vi "Event Handler.vi"(0 "uService Template in":refnum<class "Detector Manager.lvclass">, 5 "Event type":T1=enum."Message", 7 "Item Name":string, 9 "Data":variant, 11 "error in (no error)":errorcluster) -> (4 "uService Template out":refnum<class "Detector Manager.lvclass">, 15 "error out":errorcluster)   [LabVIEW 2026, in "TALOS.lvlib" / "Detector Manager.lvlib" / "Detector Manager.lvclass"]
uses:
  Detector Manager.lvclass
  C:/LabVIEW Code/TALOS/talos/Father of all uServices/Father of all uServices/Father of all uServices.lvclass
  Father of all uServices/Father of all uServices/Event Handler Items.ctl
  Ancestor/Ancestor/Ancestor.lvclass/Ancestor.ctl
  Detector Manager Consumer Case Selector.ctl
  Detector Manager.lvclass/Detector Manager.ctl
  Father of all uServices/Father of all uServices Messages/Consumer Msg/Consumer Msg.lvclass/Consumer Msg.ctl
  FGV/Error Memory/Get Error Description.vi
  Support VIs/Get PC name.vi
  Ancestor/Ancestor/Read ID.vi
  Support VIs/Get Class Name.vi
  <vilib>/Utility/error.llb/Clear Errors.vi
  Father of all uServices/Father of all uServices Messages/Consumer Msg/Send Consumer.vi
  FGV/Error Memory/Error Memory Core.vi
  <vilib>/AdvancedString/Delimited String to 1D String Array.vi
  <vilib>/AdvancedString/Delimited String to 1D String Array (string).vi
  Support VIs/Circus Root Path.vi
  FGV/Error Memory/Error Crt Lvl checker.vi
  FGV/Error Memory/Error Memory Core.vi/40c8088d-b597-4017-91af-faa98e00292e.vi
  FGV/Error Memory/Error Memory Core.vi/d4a3ab98-063c-4e44-b43d-fbdcfe6c2be2.vi
  Father of all uServices/Father of all uServices/Father of all uServices.lvclass
  C:/LabVIEW Code/TALOS/builds/Actor Framework PPL/Actor Framework.lvlibp/1abvi3w/vi.lib/ActorFramework/Actor/Actor.lvclass
  Support VIs/Global Memory.vi
  <vilib>/Utility/LVClass/Get LV Class Name.vi
  Support VIs/Is in Packed Library.vi
  Support VIs/TALOS Root path.vi
  Support VIs/Read CSV worksheet.vi
  Support VIs/Global Constants.vi
  <vilib>/Utility/error.llb/General Error Handler.vi
  builds/Actor Framework PPL/Actor Framework.lvlibp/1abvi3w/vi.lib/ActorFramework/Actor/Read Self Enqueuer.vi
  <userlib>/_OpenG.lib/lvdata/lvdata.llb/Get Strings from Enum__ogtk.vi
  builds/Actor Framework PPL/Actor Framework.lvlibp/1abvi3w/vi.lib/ActorFramework/Message Enqueuer/Enqueue.vi
  Support VIs/Error Log.vi
  Ancestor/Ancestor/Ancestor.lvclass
  <vilib>/Comparison/Equal/Equal Functor/Equal Functor.lvclass
  Father of all uServices/Father of all uServices Messages/Consumer Msg/Consumer Msg.lvclass
  Classes/Father of all Detectors/Father Of All Detectors.lvclass
  TALOS.lvlib
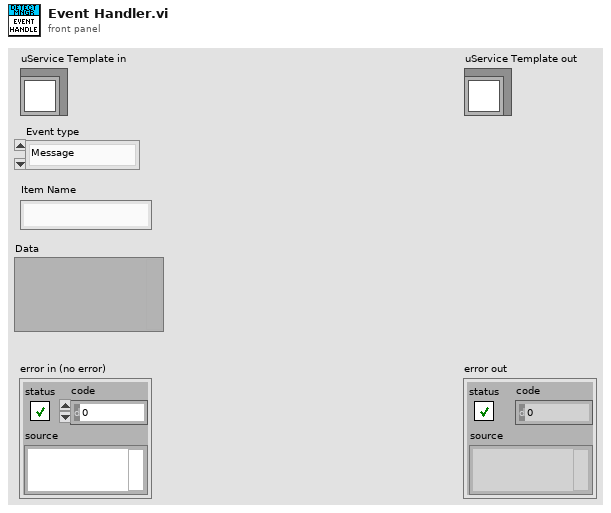
[diagram p1: front panel]
types:
  T1 = typedef "TALOS.lvlib/Father of all uServices.lvlib/Father of all uServices.lvclass/Event Handler Items.ctl" = enum16{"Button Pressed", "Message", "Ready to launch?", "Safe Mode", "Start RUN", "Stop RUN"}
  T2 = typedef "TALOS.lvlib/Detector Manager.lvlib/Detector Manager.lvclass/Detector Manager Consumer Case Selector.ctl" = enum16{"Set Configuration", "Arm", "Acquiring", "Save Data", "Self Check", "Safe Mode", "Init", "Close", "Stop"}
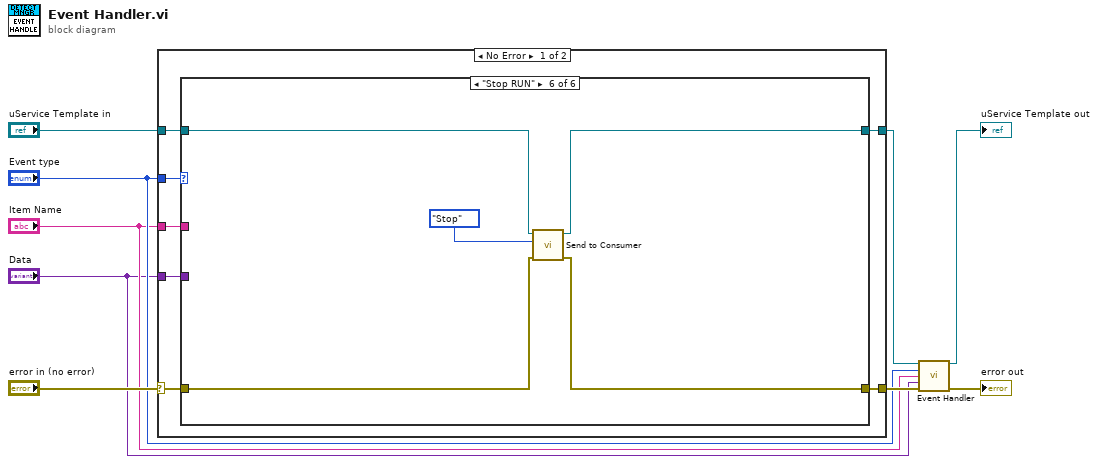
[diagram p0: block diagram]
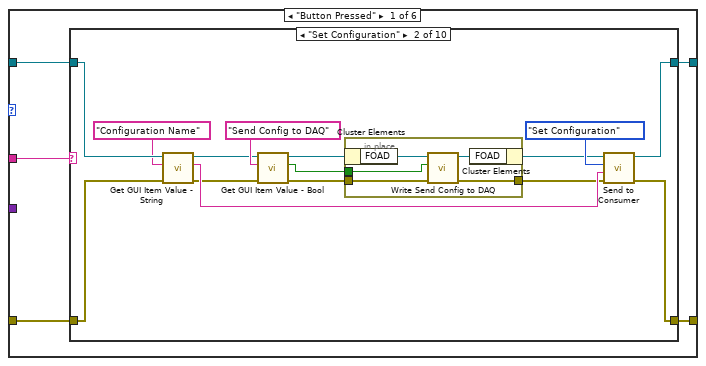
[diagram p2: hidden frame]
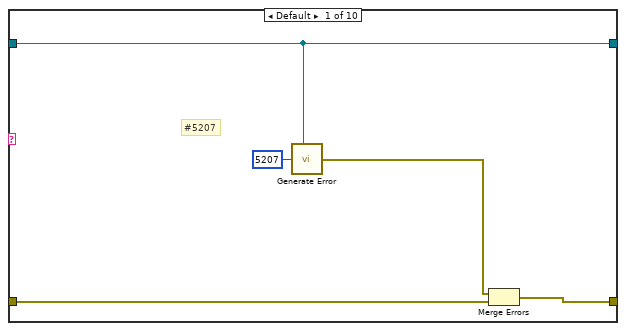
[diagram p3: hidden frame]
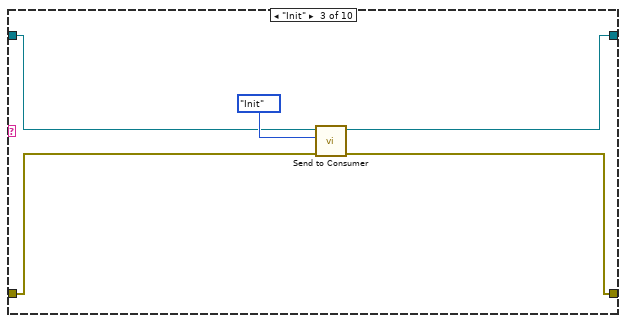
[diagram p4: hidden frame]
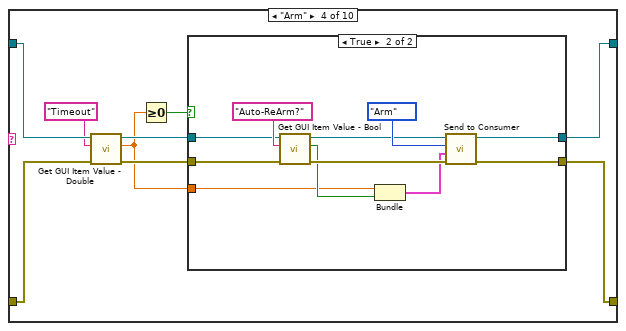
[diagram p5: hidden frame]
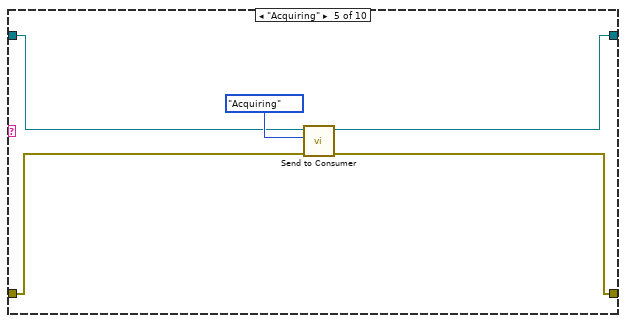
[diagram p7: hidden frame]
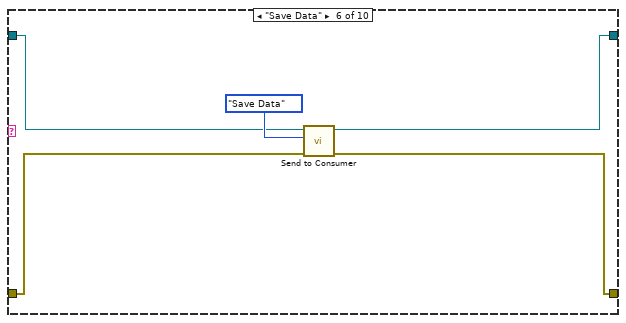
[diagram p8: hidden frame]
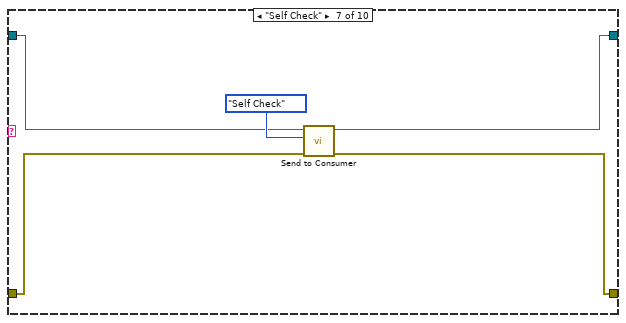
[diagram p9: hidden frame]
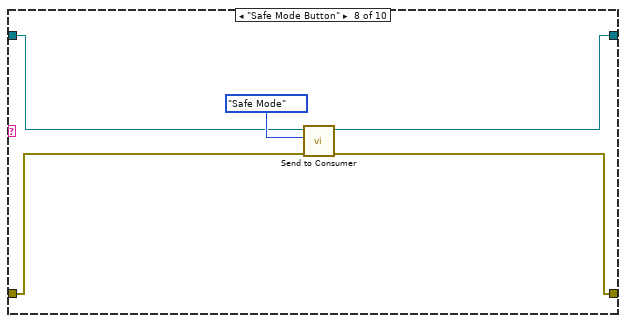
[diagram p10: hidden frame]
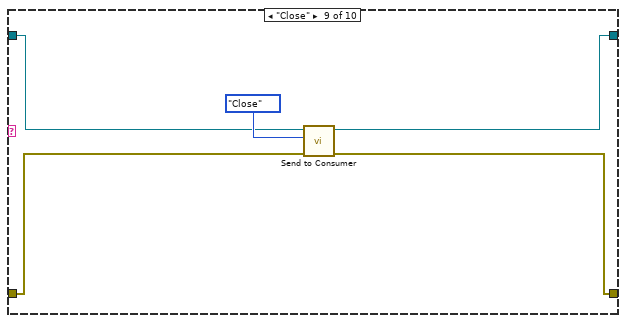
[diagram p11: hidden frame]
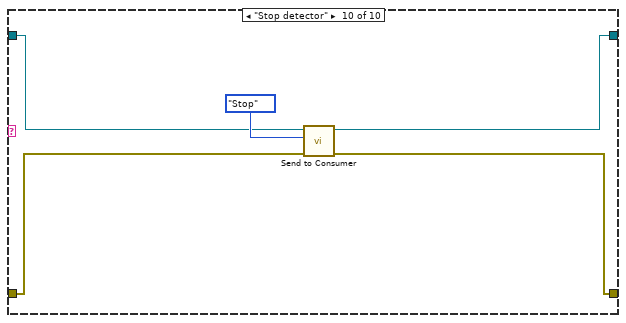
[diagram p12: hidden frame]
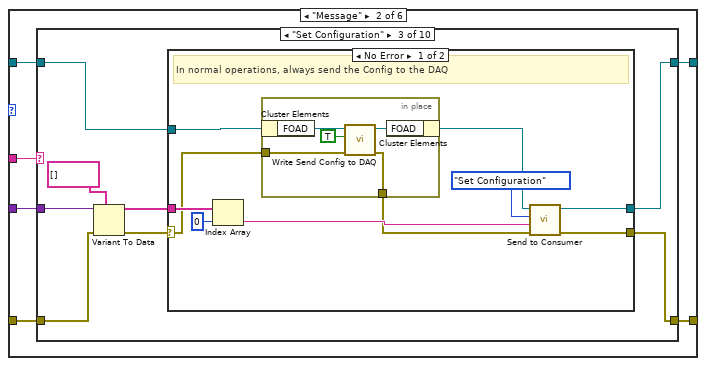
[diagram p13: hidden frame]
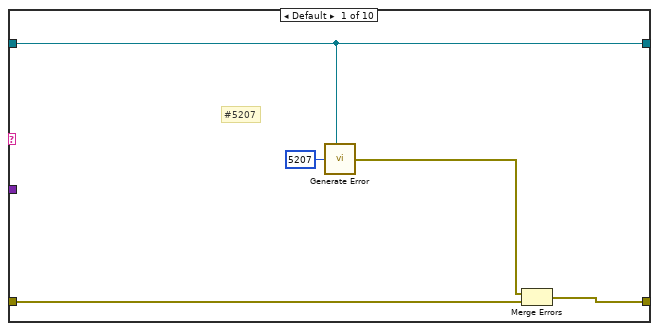
[diagram p14: hidden frame]
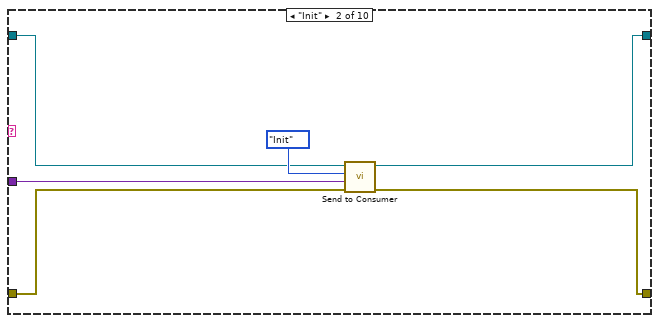
[diagram p15: hidden frame]
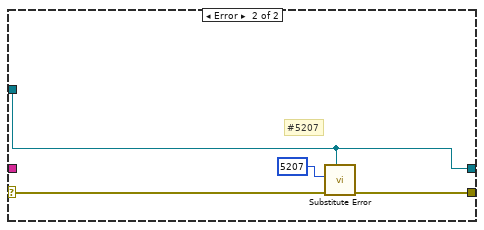
[diagram p16: hidden frame]
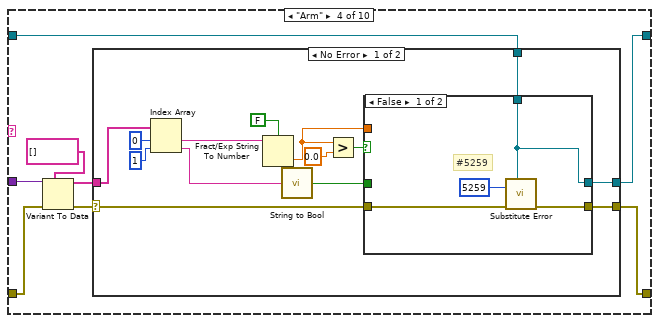
[diagram p17: hidden frame]
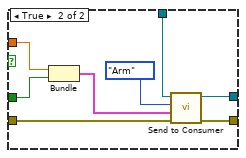
[diagram p18: hidden frame]
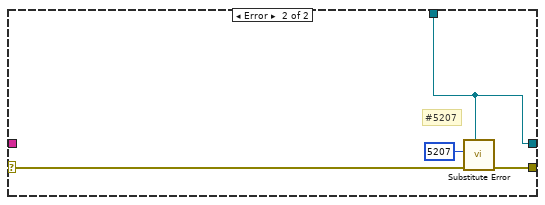
[diagram p19: hidden frame]
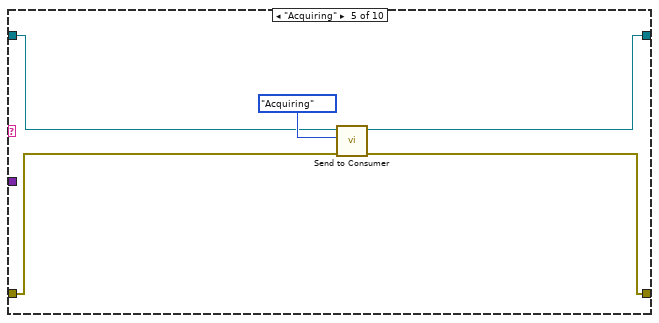
[diagram p20: hidden frame]
diagram:
  n1 = case shown="No Error" "error in (no error)" {
    selector: "error in (no error)" -> [w13 w235]
    tunnel: [w12 w235] -> w7
    tunnel: "uService Template in" -> [w15 w234]
    tunnel: [w14 w234] -> w4
    tunnel: "Event type" -> [w16 _]
    tunnel: "Item Name" -> [w11 _]
    tunnel: "Data" -> [w10 _]
    frame No Error {
      n2 = case shown="\"Stop RUN\"" w16 {
        tunnel: w15 -> [w21 w109 w220 w224 w228 w232]
        tunnel: [w20 w108 w219 w225 w228 w229] -> w14
        tunnel: w13 -> [w17 w105 w218 w222 w227 w231]
        tunnel: [w18 w106 w217 w223 w227 w230] -> w12
        tunnel: w11 -> [w19 w107 _ _ _ _]
        tunnel: w10 -> [_ w104 w216 _ _ _]
        frame "Button Pressed" {
          n3 = case shown="\"Set Configuration\"" w19 {
            tunnel: w21 -> [w22 w40 w50 w60 w77 w82 w87 w92 w97 w102]
            tunnel: [w22 w39 w49 w59 w76 w81 w86 w91 w96 w101] -> w20
            tunnel: [w25 w38 w48 w58 w75 w80 w85 w90 w95 w100] -> w18
            tunnel: w17 -> [w26 w37 w47 w57 w74 w79 w84 w89 w94 w99]
            frame Default {
              # "#5207"
              n4 = call "Generate Error.vi"("Class"=w22, "Error Code"=5207) -> ("error out"=w24:errorcluster)  [unwired: 5 in]
              n5 = Merge Errors(w24, w26) -> (w25:errorcluster)
            }
            frame "Set Configuration" {
              n6 = call "Get GUI Item Value - String.vi"("error in (no error)"=w37, "FP Item Name"="Configuration Name", "uService Template in"=w40) -> ("error out"=w33:errorcluster, "Value"=w35:string, "uService Template out"=w32:refnum<class "Detector Manager.lvclass">)  [unwired: 6 in]
              n7 = call "Get GUI Item Value - Bool.vi"("error in (no error)"=w33, "FP Item Name"="Send Config to DAQ", "uService Template in"=w32) -> ("error out"=w31:errorcluster, "Value"=w29:bool, "uService Template out"=w28:refnum<class "Detector Manager.lvclass">)  [unwired: 6 in]
              n8 = in-place {
                in-place-border: w31 -> [w44]
                in-place-border: [w43] -> w30
                in-place-border: w29 -> [w42]
                n9 = in-place-cluster #1(w28) -> ("FOAD"=w46:refnum<class "Father Of All Detectors.lvclass">)
                n10 = call-dynamic "Write Send Config to DAQ.vi"("error in (no error)"=w44, "Send Config to DAQ"=w42, "Father Of All Detectors in"=w46) -> ("error out"=w43:errorcluster, "Father Of All Detectors out"=w45:refnum<class "Father Of All Detectors.lvclass">)  [unwired: 7 in]
                n11 = in-place-cluster #1("FOAD"=w45) -> (w27:refnum<class "Detector Manager.lvclass">)
              }
              n12 = call "Send to Consumer.vi"("error in (no error)"=w30, "Data"=w35, "Case ID"=Detector_Manager_Consumer_Case_Selector."Set Configuration", "uService Template in"=w27) -> ("error out"=w38:errorcluster, "uService Template out"=w39:refnum<class "Detector Manager.lvclass">)  [unwired: 6 in]
            }
            frame "Init" {
              n13 = call "Send to Consumer.vi"("error in (no error)"=w47, "Case ID"=Detector_Manager_Consumer_Case_Selector."Init", "uService Template in"=w50) -> ("error out"=w48:errorcluster, "uService Template out"=w49:refnum<class "Detector Manager.lvclass">)  [unwired: 7 in]
            }
            frame "Arm" {
              n14 = call "Get GUI Item Value - Double.vi"("error in (no error)"=w57, "FP Item Name"="Timeout", "uService Template in"=w60) -> ("error out"=w54:errorcluster, "Value"=w53:dbl, "uService Template out"=w55:refnum<class "Detector Manager.lvclass">)  [unwired: 6 in]
              n15 = Greater Or Equal To 0?(x=w53) -> (x >= 0?=w52:bool)
              n16 = case shown="True" w52 {
                tunnel: [w62 w72] -> w59
                tunnel: [w61 w71] -> w58
                tunnel: w55 -> [w62 w69]
                tunnel: w54 -> [w61 w67]
                tunnel: w53 -> [_ w63]
                frame False {
                }
                frame True {
                  n17 = call "Get GUI Item Value - Bool.vi"("error in (no error)"=w67, "FP Item Name"="Auto-ReArm?", "uService Template in"=w69) -> ("error out"=w66:errorcluster, "Value"=w65:bool, "uService Template out"=w68:refnum<class "Detector Manager.lvclass">)  [unwired: 6 in]
                  n18 = Bundle("Value"=w63, "Value"=w65) -> (w64:cluster{"Value":dbl, "Value":bool})  [unwired: 1 in]
                  n19 = call "Send to Consumer.vi"("error in (no error)"=w66, "Data"=w64, "Case ID"=Detector_Manager_Consumer_Case_Selector."Arm", "uService Template in"=w68) -> ("error out"=w71:errorcluster, "uService Template out"=w72:refnum<class "Detector Manager.lvclass">)  [unwired: 6 in]
                }
              }
            }
            frame "Acquiring" {
              n20 = call "Send to Consumer.vi"("error in (no error)"=w74, "Case ID"=Detector_Manager_Consumer_Case_Selector."Acquiring", "uService Template in"=w77) -> ("error out"=w75:errorcluster, "uService Template out"=w76:refnum<class "Detector Manager.lvclass">)  [unwired: 7 in]
            }
            frame "Save Data" {
              n21 = call "Send to Consumer.vi"("error in (no error)"=w79, "Case ID"=Detector_Manager_Consumer_Case_Selector."Save Data", "uService Template in"=w82) -> ("error out"=w80:errorcluster, "uService Template out"=w81:refnum<class "Detector Manager.lvclass">)  [unwired: 7 in]
            }
            frame "Self Check" {
              n22 = call "Send to Consumer.vi"("error in (no error)"=w84, "Case ID"=Detector_Manager_Consumer_Case_Selector."Self Check", "uService Template in"=w87) -> ("error out"=w85:errorcluster, "uService Template out"=w86:refnum<class "Detector Manager.lvclass">)  [unwired: 7 in]
            }
            frame "Safe Mode Button" {
              n23 = call "Send to Consumer.vi"("error in (no error)"=w89, "Case ID"=Detector_Manager_Consumer_Case_Selector."Safe Mode", "uService Template in"=w92) -> ("error out"=w90:errorcluster, "uService Template out"=w91:refnum<class "Detector Manager.lvclass">)  [unwired: 7 in]
            }
            frame "Close" {
              n24 = call "Send to Consumer.vi"("error in (no error)"=w94, "Case ID"=Detector_Manager_Consumer_Case_Selector."Close", "uService Template in"=w97) -> ("error out"=w95:errorcluster, "uService Template out"=w96:refnum<class "Detector Manager.lvclass">)  [unwired: 7 in]
            }
            frame "Stop detector" {
              n25 = call "Send to Consumer.vi"("error in (no error)"=w99, "Case ID"=Detector_Manager_Consumer_Case_Selector."Stop", "uService Template in"=w102) -> ("error out"=w100:errorcluster, "uService Template out"=w101:refnum<class "Detector Manager.lvclass">)  [unwired: 7 in]
            }
          }
        }
        frame "Message" {
          n26 = case shown="\"Set Configuration\"" w107 {
            tunnel: w109 -> [w110 w116 w126 w153 w189 w194 w199 w204 w209 w214]
            tunnel: [w110 w119 w128 w155 w188 w193 w198 w203 w208 w213] -> w108
            tunnel: [w113 w118 w127 w154 w187 w192 w197 w202 w207 w212] -> w106
            tunnel: w105 -> [w114 w117 w121 w149 w186 w191 w196 w201 w206 w211]
            tunnel: w104 -> [_ w115 w125 w152 _ _ _ _ _ _]
            frame Default {
              # "#5207"
              n27 = call "Generate Error.vi"("Class"=w110, "Error Code"=5207) -> ("error out"=w112:errorcluster)  [unwired: 5 in]
              n28 = Merge Errors(w112, w114) -> (w113:errorcluster)
            }
            frame "Init" {
              n29 = call "Send to Consumer.vi"("error in (no error)"=w117, "Data"=w115, "Case ID"=Detector_Manager_Consumer_Case_Selector."Init", "uService Template in"=w116) -> ("error out"=w118:errorcluster, "uService Template out"=w119:refnum<class "Detector Manager.lvclass">)  [unwired: 6 in]
            }
            frame "Set Configuration" {
              n30 = Variant To Data(error in=w121, type=string[] [], Variant=w125) -> (data=w123:string[], error out=w122:errorcluster)
              n31 = case shown="No Error" w122 {
                selector: w122 -> [w130 w144]
                tunnel: [w137 w146] -> w128
                tunnel: [w136 w145] -> w127
                tunnel: w126 -> [w132 w146]
                tunnel: w123 -> [w133 _]
                frame No Error {
                  # "In normal operations, always send the Config to the DAQ"
                  n32 = Index Array(array=w133, index=0) -> (element=w134:string)
                  n33 = in-place {
                    in-place-border: w130 -> [w141]
                    in-place-border: [w140] -> w129
                    n34 = in-place-cluster #2(w132) -> ("FOAD"=w143:refnum<class "Father Of All Detectors.lvclass">)
                    n35 = call-dynamic "Write Send Config to DAQ.vi"("error in (no error)"=w141, "Send Config to DAQ"=TRUE, "Father Of All Detectors in"=w143) -> ("error out"=w140:errorcluster, "Father Of All Detectors out"=w142:refnum<class "Father Of All Detectors.lvclass">)  [unwired: 7 in]
                    n36 = in-place-cluster #2("FOAD"=w142) -> (w131:refnum<class "Detector Manager.lvclass">)
                  }
                  n37 = call "Send to Consumer.vi"("error in (no error)"=w129, "Data"=w134, "Case ID"=Detector_Manager_Consumer_Case_Selector."Set Configuration", "uService Template in"=w131) -> ("error out"=w136:errorcluster, "uService Template out"=w137:refnum<class "Detector Manager.lvclass">)  [unwired: 6 in]
                }
                frame Error {
                  # "#5207"
                  n38 = call "Substitute Error.vi"("LabVIEW Object"=w146, "error in (no error)"=w144, "Error Code"=5207) -> ("error out"=w145:errorcluster)  [unwired: 8 in]
                }
              }
            }
            frame "Arm" {
              n39 = Variant To Data(error in=w149, type=string[] [], Variant=w152) -> (data=w151:string[], error out=w150:errorcluster)
              n40 = case shown="No Error" w150 {
                selector: w150 -> [w160 w182]
                tunnel: [w156 w184] -> w155
                tunnel: [w157 w185] -> w154
                tunnel: w153 -> [w158 w184]
                tunnel: w151 -> [w161 _]
                frame No Error {
                  n41 = Index Array(array=w161, index #1=0 ("index"), index #2=1 ("index")) -> (element #1=w168:string, element #2=w162:string)
                  n42 = Fract/Exp String To Number(use system decimal point (T)=FALSE, string=w168) -> (number=w164:dbl)  [unwired: 2 in, 1 out]
                  n43 = call "String to Bool.vi"("String"=w162) -> ("Boolean"=w159:bool)
                  n44 = Greater?(x=w164, y=0.0) -> (0:w165:bool)
                  n45 = case shown="False" w165 {
                    tunnel: w160 -> [w172 w176]
                    tunnel: w164 -> [_ w181]
                    tunnel: w159 -> [_ w180]
                    tunnel: w158 -> [w170 w179]
                    tunnel: [w173 w178] -> w157
                    tunnel: [w170 w177] -> w156
                    frame False {
                      # "#5259"
                      n46 = call "Substitute Error.vi"("LabVIEW Object"=w170, "error in (no error)"=w172, "Error Code"=5259) -> ("error out"=w173:errorcluster)  [unwired: 8 in]
                    }
                    frame True {
                      n47 = Bundle(w181, "Boolean"=w180) -> (w174:cluster{dbl, "Boolean":bool})  [unwired: 1 in]
                      n48 = call "Send to Consumer.vi"("error in (no error)"=w176, "Data"=w174, "Case ID"=Detector_Manager_Consumer_Case_Selector."Arm", "uService Template in"=w179) -> ("error out"=w178:errorcluster, "uService Template out"=w177:refnum<class "Detector Manager.lvclass">)  [unwired: 6 in]
                    }
                  }
                }
                frame Error {
                  # "#5207"
                  n49 = call "Substitute Error.vi"("LabVIEW Object"=w184, "error in (no error)"=w182, "Error Code"=5207) -> ("error out"=w185:errorcluster)  [unwired: 8 in]
                }
              }
            }
            frame "Acquiring" {
              n50 = call "Send to Consumer.vi"("error in (no error)"=w186, "Case ID"=Detector_Manager_Consumer_Case_Selector."Acquiring", "uService Template in"=w189) -> ("error out"=w187:errorcluster, "uService Template out"=w188:refnum<class "Detector Manager.lvclass">)  [unwired: 7 in]
            }
            frame "Save Data" {
              n51 = call "Send to Consumer.vi"("error in (no error)"=w191, "Case ID"=Detector_Manager_Consumer_Case_Selector."Save Data", "uService Template in"=w194) -> ("error out"=w192:errorcluster, "uService Template out"=w193:refnum<class "Detector Manager.lvclass">)  [unwired: 7 in]
            }
            frame "Self Check" {
              n52 = call "Send to Consumer.vi"("error in (no error)"=w196, "Case ID"=Detector_Manager_Consumer_Case_Selector."Self Check", "uService Template in"=w199) -> ("error out"=w197:errorcluster, "uService Template out"=w198:refnum<class "Detector Manager.lvclass">)  [unwired: 7 in]
            }
            frame "Safe Mode" {
              n53 = call "Send to Consumer.vi"("error in (no error)"=w201, "Case ID"=Detector_Manager_Consumer_Case_Selector."Safe Mode", "uService Template in"=w204) -> ("error out"=w202:errorcluster, "uService Template out"=w203:refnum<class "Detector Manager.lvclass">)  [unwired: 7 in]
            }
            frame "Close" {
              n54 = call "Send to Consumer.vi"("error in (no error)"=w206, "Case ID"=Detector_Manager_Consumer_Case_Selector."Close", "uService Template in"=w209) -> ("error out"=w207:errorcluster, "uService Template out"=w208:refnum<class "Detector Manager.lvclass">)  [unwired: 7 in]
            }
            frame "Stop" {
              n55 = call "Send to Consumer.vi"("error in (no error)"=w211, "Case ID"=Detector_Manager_Consumer_Case_Selector."Stop", "uService Template in"=w214) -> ("error out"=w212:errorcluster, "uService Template out"=w213:refnum<class "Detector Manager.lvclass">)  [unwired: 7 in]
            }
          }
        }
        frame "Ready to launch?" {
          n56 = call "Send to Consumer.vi"("error in (no error)"=w218, "Data"=w216, "Case ID"=Detector_Manager_Consumer_Case_Selector."Self Check", "uService Template in"=w220) -> ("error out"=w217:errorcluster, "uService Template out"=w219:refnum<class "Detector Manager.lvclass">)  [unwired: 6 in]
        }
        frame "Safe Mode" {
          n57 = call "Send to Consumer.vi"("error in (no error)"=w222, "Case ID"=Detector_Manager_Consumer_Case_Selector."Safe Mode", "uService Template in"=w224) -> ("error out"=w223:errorcluster, "uService Template out"=w225:refnum<class "Detector Manager.lvclass">)  [unwired: 7 in]
        }
        frame "Start RUN" {
        }
        frame "Stop RUN" {
          n58 = call "Send to Consumer.vi"("error in (no error)"=w231, "Case ID"=Detector_Manager_Consumer_Case_Selector."Stop", "uService Template in"=w232) -> ("error out"=w230:errorcluster, "uService Template out"=w229:refnum<class "Detector Manager.lvclass">)  [unwired: 7 in]
        }
      }
    }
    frame Error {
    }
  }
  n59 = call-parent "Event Handler.vi"("uService Template in"=w4, "Event type"="Event type", "Item Name"="Item Name", "Data"="Data", "error in (no error)"=w7) -> ("uService Template out"=→"uService Template out":refnum<class "Detector Manager.lvclass">, "error out"=→"error out":errorcluster)  [unwired: 9 in]
